vi "MT_write_old.vi"(6 "stop":bool, 7 "Physical Channels":tag, 8 "error in":errorcluster, 9 "duration":dbl, 10 "signal":dbl[](array[numeric]), 11 "sampling rate":dbl) -> (0 "error out":errorcluster)   [LabVIEW 2019]
uses:
  <vilib>/DAQmx/write.llb/DAQmx Write (Analog 1D DBL 1Chan NSamp).vi
  <vilib>/DAQmx/create/channels.llb/DAQmx Create Channel (AO-Voltage-Basic).vi
  <vilib>/DAQmx/configure/timing.llb/DAQmx Timing (Sample Clock).vi
  <vilib>/DAQmx/miscellaneous.llb/DAQmx Fill In Error Info.vi
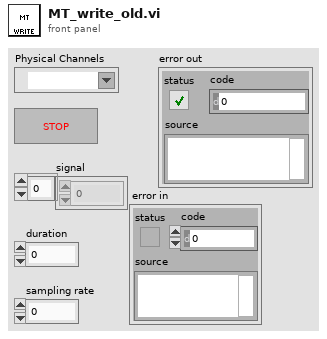
[diagram p1: front panel]
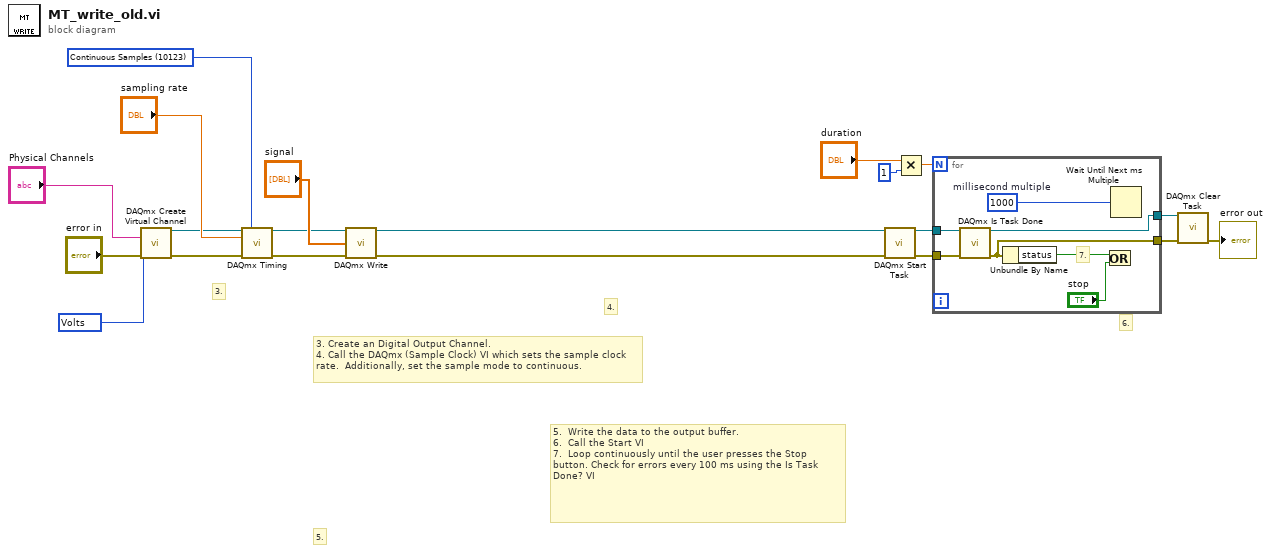
[diagram p0: block diagram]
diagram:
  w1 = 10348 items=["Volts"=10348, "From Custom Scale"=10065] ("units")
  w5 = 10123 items=["Finite Samples"=10178, "Continuous Samples"=10123] ("sample mode")
  # "6."
  # "5."
  # "5.  Write the data to the output buffer.\n6.  Call the Start VI\n7.  Loop continuously until the user presses the Stop button. Check for errors every 100 ms using the Is Task Done? VI"
  # "4."
  # "3. Create an Digital Output Channel. \n4. Call the DAQmx (Sample Clock) VI which sets the sample clock rate.  Additionally, set the sample mode to continuous."
  # "3."
  n1 = call-poly <vilib>:"DAQmx Create Virtual Channel.vi"("physical channels"="Physical Channels", "units"=w1, "error in"="error in") -> ("task out"=w11:refnum<k21>, "error out"=w12:errorcluster)  [unwired: 6 in, 5 out]
  n2 = call-poly <vilib>:"DAQmx Timing.vi"("task/channels in"=w11, "sample mode"=w5, "rate"="sampling rate", "error in"=w12) -> ("task out"=w13:refnum<k21>, "error out"=w14:errorcluster)  [unwired: 3 in, 7 out]
  n3 = call-poly <vilib>:"DAQmx Write.vi"("task/channels in"=w13, "data"="signal", "error in"=w14) -> ("task out"=w6:refnum<k21>, "error out"=w7:errorcluster)  [unwired: 1 in, 10 out]
  n4 = call <vilib>:"DAQmx Start Task.vi"("task/channels in"=w6, "error in"=w7) -> ("task out"=w4:refnum<k21>, "error out"=w8:errorcluster)  [unwired: 12 out]
  n5 = Multiply(x="duration", y=1) -> (x*y=w17:dbl)
  n6 = for {
    N: w17 -> [_]
    tunnel: w4 -> [w27]
    tunnel: [w26] -> w9
    tunnel: w8 -> [w25]
    tunnel: [w23] -> w10
    w21 = u32 1000  # millisecond multiple
    # "7."
    n7 = call <vilib>:"DAQmx Is Task Done.vi"("task/channels in"=w27, "error in"=w25) -> ("task out"=w26:refnum<k21>, "error out"=w23:errorcluster)  [unwired: 1 in, 11 out]
    n8 = Unbundle By Name(w23) -> ("status"=w24:bool)
    n9 = Or(x=w24, y="stop") -> ()  [unwired: 1 out]
    n10 = Wait Until Next ms Multiple(millisecond multiple=w21) -> ()  [unwired: 1 out]
  }
  n11 = call <vilib>:"DAQmx Clear Task.vi"("task in"=w9, "error in"=w10) -> ("error out"=→"error out":errorcluster)  [unwired: 13 out]
